vi "test.vi"() -> ()   [LabVIEW 2015]
uses:
  picoquant_Tmodes.ctl
  picoquant_devices.ctl
panel:
  out "error out":errorcluster
  in  "error in (no error)":errorcluster
  out "ch2_tally":u64
  out "ch1_tally":u64
  out "times":u64[](array[numeric])
  out "channels 2":u8[](array[numeric])
  out "ch2_array":u64[](array[numeric])
  out "ch1_array":u64[](array[numeric])
  out "32bit integer":i32
  out "max value":u64
  in  "Device":T1
  in  "acq_mode":T2=2 items=["T2"=2, "T3"=3]
  out "photon_count":u64
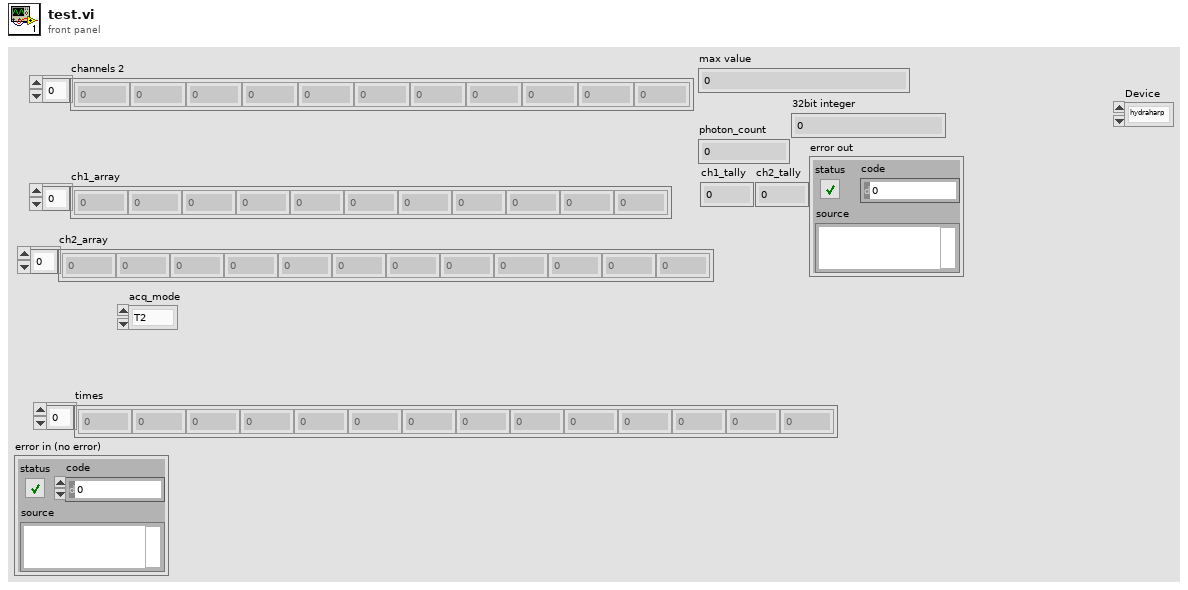
[diagram p1: front panel]
types:
  T1 = typedef "picoquant_devices.ctl" = enum16{"hydraharp", "picoharp"}
  T2 = typedef "picoquant_Tmodes.ctl" = u16
  T3 = enum16{"big-endian, network order", "native, host order", "little-endian"}
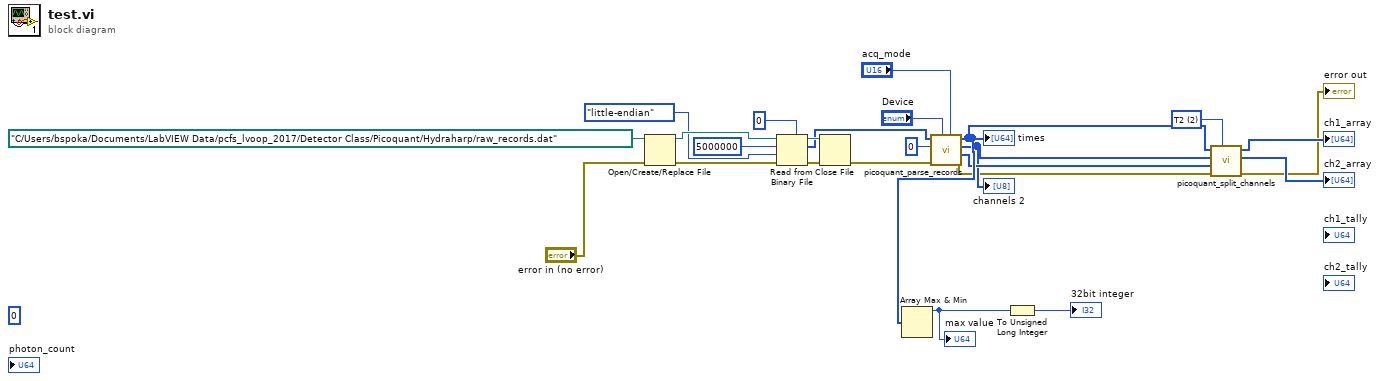
[diagram p0: block diagram]
diagram:
  w1 = T2 2 items=["T2"=2, "T3"=3] ("acq_mode")
  (unwired) u64 0 ("overflow")
  n1 = Open/Create/Replace File(file path (use dialog)=path "C:/Users/bspoka/Documents/LabVIEW Data/pcfs_lvoop_2017/Detector Class/Picoquant/Hydraharp/raw_records.dat", error in="error in (no error)") -> (refnum out=w23:refnum<file>, error out=w22:errorcluster)  [unwired: 4 in, 1 out]
  n2 = Read from Binary File(5:u32 0, 8:w22, 9:T3."little-endian" ("byte order (0:big-endian, network order)"), 10:5000000 ("count (1)"), 11:w23) -> (0:w20:errorcluster, 2:w5:u32[], 3:w21:refnum<file>)  [unwired: 1 in, 1 out]
  n3 = Close File(refnum=w21, error in=w20) -> (error out=w7:errorcluster)  [unwired: 1 out]
  n4 = call "picoquant_parse_records.vi"("acq_mode"="acq_mode", "Device"="Device", "error in (no error)"=w7, "overflow"=u64 0, "fifo_buffer"=w5) -> ("error out"=w3:errorcluster, "sync"=w11:u64[], "channels"=w10:u8[], "times"=w12:u64[])  [unwired: 1 in, 2 out]
  "channels 2" <- w10
  "times" <- w12
  n5 = Array Max & Min(array=w12) -> (max value=w13:u64)  [unwired: 3 out]
  "max value" <- w13
  n6 = To Unsigned Long Integer(number=w13) -> (unsigned 32bit integer=→"32bit integer":u32)
  n7 = call "picoquant_split_channels.vi"("acq_mode"=w1, "error in (no error)"=w3, "sync"=w11, "channels"=w10, "times"=w12) -> ("error out"=→"error out":errorcluster, "ch2_array"=→"ch2_array":u64[], "ch1_array"=→"ch1_array":u64[])  [unwired: 2 in, 2 out]
